vi "Chi-Squared Inverse CDF.vi"(10 "k":i32=1, 11 "cdf(x)":dbl=0.682689492137086) -> (0 "error":i32, 3 "x":dbl=1.0)   [LabVIEW 2018, in "NI_Gmath.lvlib"]
doc: "Computes the continuous inverse cumulative distribution function (CDF) of the various distributions. You must manually select the polymorphic instance to use."
uses:
  NI_Gmath.lvlib
  st_error_code.ctl
panel:
  # "Chi-Squared Inverse CDF"
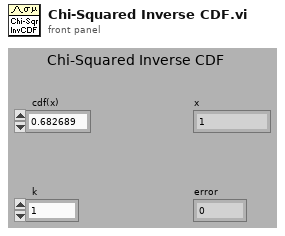
[diagram p1: front panel]
types:
  T1 = typedef "NI_Gmath.lvlib/st_error_code.ctl" = i32
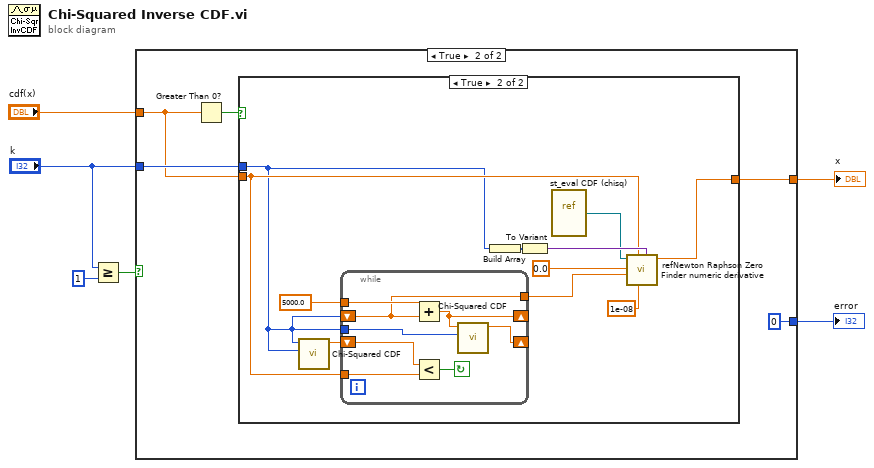
[diagram p0: block diagram]
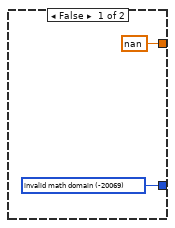
[diagram p2: hidden frame]
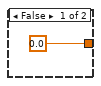
[diagram p3: hidden frame]
diagram:
  n1 = Greater Or Equal?(x="k", y=1) -> (x >= y?=w1:bool)
  n2 = case shown="True" w1 {
    tunnel: [w7 0 ("invalid math domain")] -> w6
    tunnel: [nan w12] -> w5
    tunnel: "cdf(x)" -> [_ w10]
    tunnel: "k" -> [_ w11]
    frame False {
      w7 = T1 -20069 items=["invalid math domain"=-20069, "Fourier interpolation size m >= n"=-20070, "empty array"=-20003] ("stat interp error code")
    }
    frame True {
      n3 = Greater Than 0?(x=w10) -> (x > 0?=w9:bool)
      n4 = case shown="True" w9 {
        tunnel: [0.0 w24] -> w12
        tunnel: w10 -> [_ w18]
        tunnel: w11 -> [_ w15]
        frame False {
        }
        frame True {
          n5 = call "Chi-Squared CDF.vi"("k"=w15, "x"=w15) -> ("cdf(x)"=w19:dbl)  [unwired: 8 in, 1 out]
          n6 = while {
            shift-right: [w30] -> _
            shift-left: w19 -> [w32]
            tunnel: w18 -> [w31]
            shift-right: [w28] -> _
            shift-left: w15 -> [w26]
            tunnel: w15 -> [w29]
            tunnel: 5000.0 ("upper limit") -> [w27]
            tunnel: [w26] -> w16
            stop <- w33 continue-if-true
            n7 = Add(x=w27, y=w26) -> (x+y=w28:dbl)
            n8 = Less?(x=w32, y=w31) -> (x < y?=w33:bool)
            n9 = call "Chi-Squared CDF.vi"("k"=w29, "x"=w28) -> ("cdf(x)"=w30:dbl)  [unwired: 8 in, 1 out]
          }
          n10 = Build Array(w15) -> (w25:i32[])
          n11 = To Variant(anything=w25) -> (Variant=w23:variant)
          n12 = vi-ref "st_eval CDF (chisq).vi"() -> ("vi reference"=w22:refnum<vi>)
          n13 = call "refNewton Raphson Zero Finder numeric derivative.vi"("function parameters"=w23, "accuracy"=1e-08, "level"=w18, "end"=w16, "start"=0.0 ("upper limit"), "function refnum"=w22) -> ("zero"=w24:dbl)  [unwired: 2 in, 3 out]
        }
      }
    }
  }
  "x" <- w5
  "error" <- w6
